vi "Create Image from ROI_LV_2009.vi"() -> ()   [LabVIEW 2015]
uses:
  <vilib>/vision/NI_Vision_Development_Module.lvlib
panel:
  in  "Rectangle":T1 {"Rotation" format="%.2f"; "Left" scale=0.0..1024.0; "Right" scale=0.0..1024.0}
  out "Destination Image":T2(plugin-control)
  in  "Destination Image Types":T3 items=["Grayscale (U8)", "Grayscale (I16)", "Grayscale (SGL)", "Complex (CSG)", "RGB (U32)", "HSL (U32)", "RGB (U64)", "Grayscale (U16)"]
  in  "Destination Images Folder Path":path
  out "Source Image":T2(plugin-control)
  in  "Number of Images":i32
  in  "Source Image Type":T3 items=["Grayscale (U8)", "Grayscale (I16)", "Grayscale (SGL)", "Complex (CSG)", "RGB (U32)", "HSL (U32)", "RGB (U64)", "Grayscale (U16)"]
  in  "Source Image Path":path
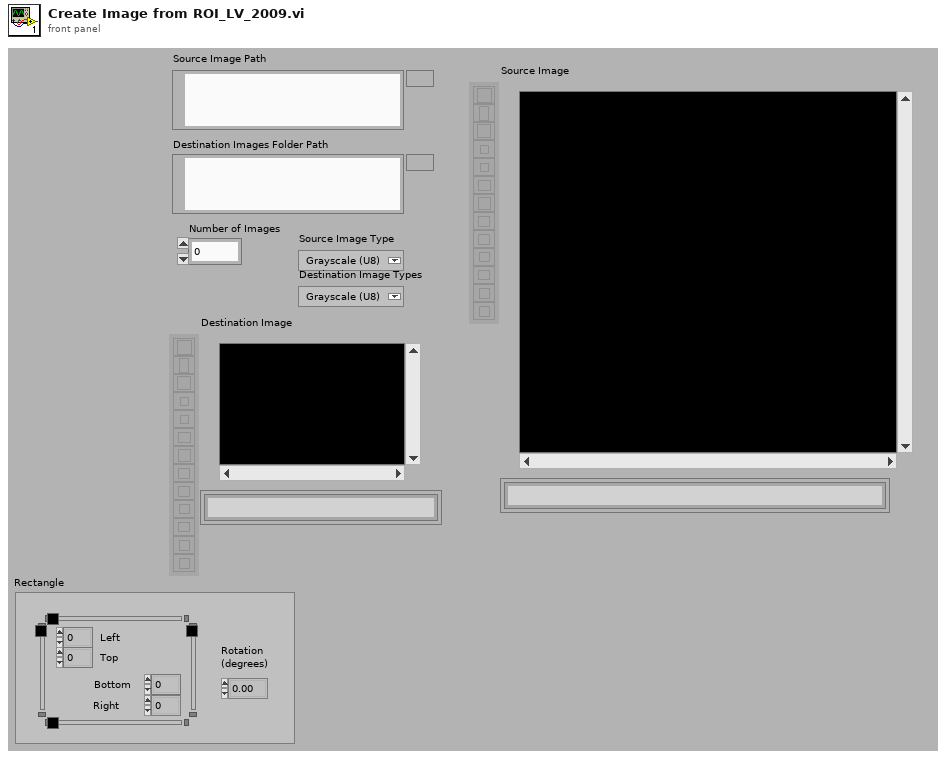
[diagram p1: front panel]
types:
  T1 = typedef "IMAQ Rectangle" = cluster{"Left":i32, "Top":i32, "Right":i32, "Bottom":i32, "Rotation":dbl}
  T2 = typedef "IMAQ Image.ctl" = refnum<image>
  T3 = typedef "Image Type" = u32
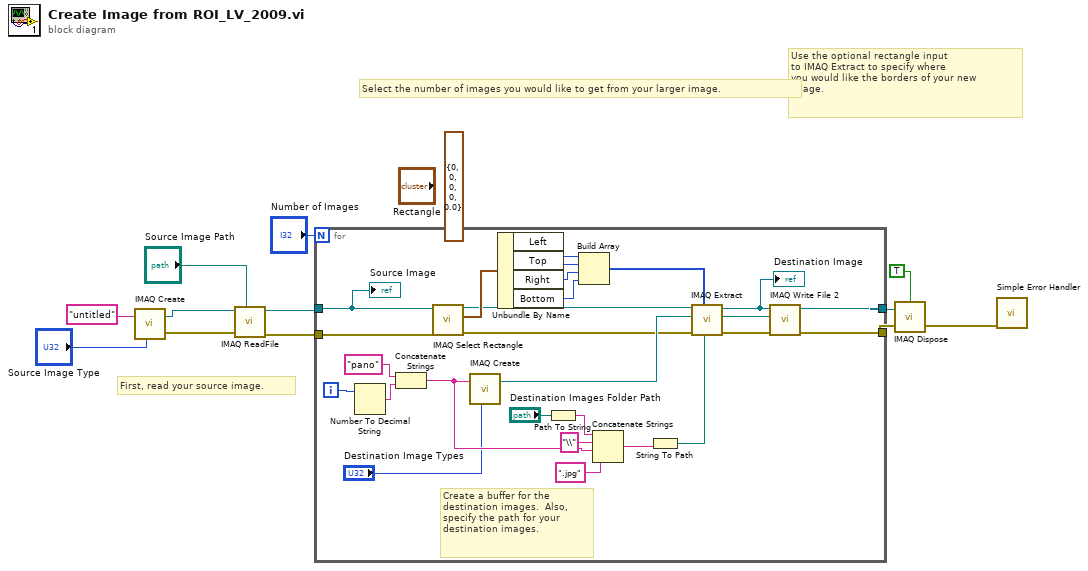
[diagram p0: block diagram]
diagram:
  (unwired) T1 {"Left"=0, "Top"=0, "Right"=0, "Bottom"=0, "Rotation"=0.0} ("Rectangle")
  # "Use the optional rectangle input \nto IMAQ Extract to specify where \nyou would like the borders of your new\nimage."
  # "Select the number of images you would like to get from your larger image."
  # "First, read your source image."
  n1 = call "IMAQ Create"("Image Name"="untitled", "Image Type"="Source Image Type") -> ("New Image"=w11:T2, "error out"=w10:errorcluster)  [unwired: 3 in]
  n2 = call "IMAQ ReadFile"("File Path"="Source Image Path", "error in (no error)"=w10, "Image"=w11) -> ("error out"=w4:errorcluster, "Image Out"=w2:T2)  [unwired: 4 in, 3 out]
  n3 = for {
    N: "Number of Images" -> [_]
    tunnel: w2 -> [w13]
    tunnel: [w35] -> w9
    tunnel: [w34] -> w8
    tunnel: w4 -> [w14]
    i -> [w36]
    # "Create a buffer for the \ndestination images.  Also,\nspecify the path for your \ndestination images."
    n4 = Number To Decimal String(number=w36) -> (decimal integer string=w37:string)  [unwired: 1 in]
    n5 = Concatenate Strings("pano", w37) -> (w28:string)
    n6 = call "IMAQ Select Rectangle"("error in (no error)"=w14, "Image In"=w13) -> ("error out"=w16:errorcluster, "Rectangle"=w25:T1, "Image Out (duplicate)"=w15:T2)  [unwired: 6 in, 1 out]
    n7 = call "IMAQ Create"("Image Name"=w28, "Image Type"="Destination Image Types") -> ("New Image"=w19:T2)  [unwired: 3 in, 1 out]
    n8 = Unbundle By Name(w25) -> ("Left"=w24:i32, "Top"=w23:i32, "Right"=w22:i32, "Bottom"=w21:i32)
    n9 = Path To String(path="Destination Images Folder Path") -> (string=w32:string)
    n10 = Build Array(w24, w23, w22, w21) -> (w20:i32[])
    n11 = Concatenate Strings(w32, "\\" ("string"), w28, ".jpg" ("string")) -> (w31:string)
    n12 = String To Path(string=w31) -> (path=w30:path)
    n13 = call "IMAQ Extract"("Optional Rectangle"=w20, "error in (no error)"=w16, "Image Dst"=w19, "Image Src"=w15) -> ("error out"=w17:errorcluster, "Image Dst Out"=w18:T2)  [unwired: 6 in]
    "Destination Image" <- w18
    n14 = call-poly "IMAQ Write File 2"("error in (no error)"=w17, "File Path"=w30, "Image"=w18) -> ("error out"=w35:errorcluster, "Image Out (duplicate)"=w34:T2)  [unwired: 7 in]
    "Source Image" <- w13
  }
  n15 = call "IMAQ Dispose"("All Images? (No)"=TRUE, "Image"=w8, "error in (no error)"=w9) -> ("error out"=w6:errorcluster)  [unwired: 3 in]
  n16 = call <vilib>:"Simple Error Handler.vi"("error in (no error)"=w6) -> ()  [unwired: 4 in, 5 out]
